vi "HFRR ADV v011 new software.vi"() -> ()   [LabVIEW 2025] (continued)
        n3525 = Unbundle By Name(w4415) -> ("Heave COM Status 2"=→"COM Status" →"Instrument Status":bool, "Error Heave"=→"Error":errorcluster)  [unwired: 1 out]
        n3526 = Bundle By Name(cluster=w4415, "LastCom"=w4413) -> (w4414:T18)
      }
      frame "MAIN" {
        n3527 = Unbundle By Name(w4438) -> ("Com Port 2"=w4450:refnum<visa-resource-name>)
        n3528 = local write "Com Port 4"(w4450) -> ()
        n3529 = local read "C3 :"() -> (w4436:refnum<visa-resource-name>)
        n3530 = Bundle By Name(cluster=w4438, "Heave and Surge COM Port:"=w4436) -> (w4437:T18)
        n3531 = Equal?(x=w4450, y=w4436) -> (x = y?=w4449:bool)
        n3532 = case shown="True" w4449 {
          tunnel: [w4454 w4471] -> w4448
          tunnel: w4439 -> [w4455 w4477]
          tunnel: w4437 -> [w4453 w4475]
          tunnel: [w4452 w4470] -> w4445
          frame False {
            n3533 = call <vilib>:"Clear Errors.vi"("error in (no error)"=w4455) -> ("error out"=w4451:errorcluster)  [unwired: 5 in, 1 out]
            n3534 = call "Instrument fgv.vi"("Enum"=T30."ERROR INIT", "error in (no error) 2"=w4451, "INPUT"=w4453) -> ("error"=w4457:errorcluster, "output"=w4452:T18)  [unwired: 6 in, 1 out]
            n3535 = call <vilib>:"Clear Errors.vi"("error in (no error)"=w4457) -> ("error out"=w4454:errorcluster)  [unwired: 5 in, 1 out]
          }
          frame True {
            n3536 = call "Instrument fgv.vi"("Enum"=T30."READ", "error in (no error) 2"=w4477, "INPUT"=w4475) -> ("error"=w4476:errorcluster, "output"=w4467:T18)  [unwired: 6 in, 1 out]
            n3537 = Bundle By Name(cluster=w4467, "String 36"="String 11") -> (w4466:T18)
            n3538 = case shown="True" "Write S" {
              selector: "Write S" -> [_ w4497]
              tunnel: w4476 -> [w4490 w4496]
              tunnel: [w4490 w4495] -> w4463
              tunnel: w4466 -> [w4489 w4492]
              tunnel: [w4489 w4491] -> w4462
              frame False {
              }
              frame True {
                n3539 = Not(x=w4497) -> (.not. x?=w4493:bool)
                n3540 = local write "Write S"(w4493) -> ()
                n3541 = call "Instrument fgv.vi"("Enum"=T30."MANUAL WRITE", "error in (no error) 2"=w4496, "INPUT"=w4492) -> ("error"=w4495:errorcluster, "output"=w4491:T18)  [unwired: 6 in, 1 out]
              }
            }
            n3542 = Array Size(array="WriteHumidity") -> (size(s)=w4460:i32)
            n3543 = Greater Than 0?(x=w4460) -> (x > 0?=w4458:bool)
            n3544 = call "Instrument fgv.vi"("Enum"=T30."WRITE", "error in (no error) 2"=w4463, "WriteCC1"="WriteHumidity", "INPUT"=w4462) -> ("error"=w4473:errorcluster, "WriteCC1 2"=w4461:string[], "output"=w4472:T18)  [unwired: 5 in]
            n3545 = case shown="True" w4458 {
              tunnel: w4461 -> [_ w4479]
              frame False {
              }
              frame True {
                n3546 = local write "WriteHumidity"(w4479) -> ()
              }
            }
            n3547 = case shown="Error" w4473 {
              selector: w4473 -> [w4480 w4483]
              tunnel: w4472 -> [w4481 w4488]
              tunnel: [w4481 w4487] -> w4470
              tunnel: [w4480 w4485] -> w4471
              frame No Error {
              }
              frame Error {
                n3548 = call <vilib>:"Clear Errors.vi"("error in (no error)"=w4483) -> ("error out"=w4482:errorcluster)  [unwired: 5 in, 1 out]
                n3549 = call "Instrument fgv.vi"("Enum"=T30."ERROR INIT", "error in (no error) 2"=w4482, "INPUT"=w4488) -> ("error"=w4486:errorcluster, "output"=w4487:T18)  [unwired: 6 in, 1 out]
                n3550 = call <vilib>:"Clear Errors.vi"("error in (no error)"=w4486) -> ("error out"=w4485:errorcluster)  [unwired: 5 in, 1 out]
              }
            }
            n3551 = Unbundle By Name(w4470) -> ("LastCom"=→"LastCom":string, "Read Heave and Surge"=→"Read Humidity":string)
          }
        }
        n3552 = Unbundle By Name(w4445) -> ("Heave COM Status 2"=w4447:bool, "Heave COM Status"=w4446:bool, "Error Heave"=w4443:errorcluster, "Bytes at Heave Port"=→"Bytes at Humidity Port":dbl)
        n3553 = Unbundle By Name(w4443) -> ("status"=→"Humidity Port":bool)
        n3554 = Not(x=w4446) -> (.not. x?=w4440:bool)
        n3555 = local write "Error"(w4443) -> ()
        n3556 = Not(x=w4447) -> (.not. x?=w4441:bool)
        n3557 = local write "Instrument Status"(w4440) -> ()
        n3558 = local write "COM Status"(w4441) -> ()
        n3559 = local read "Quit"() -> (w4433:bool)
        n3560 = Select(t=enum16{"init", "MAIN", "Panel Close"}."Panel Close", s=w4433, f=enum16{"init", "MAIN", "Panel Close"}."MAIN") -> (s? t:f=w4432:enum16{"init", "MAIN", "Panel Close"})
      }
      frame "Panel Close" {
      }
      frame Default {
      }
    }
  }
  n3561 = while {
    stop <- w4528 stop-if-true
    n3562 = local read "Read Humidity"() -> (w4509:string)
    n3563 = call <vilib>:"High Resolution Polling Wait.vi"("seconds to wait"=0.1) -> ()  [unwired: 10 in, 1 out]
    n3564 = Spreadsheet String To Array(delimiter (Tab)=",", format string="", spreadsheet string=w4509, array type (2D Dbl)=string[] []) -> (array=w4523:string[])
    n3565 = for {
      tunnel: w4523 -> [w4533] mode=indexing
      tunnel: string[] ["STATE;", "SET;", "RH;", "T;", "AMB_RH;", "AMB_T;", "PUMP;", "FAN_IN;", "FAN_OUT;", "DEHUM;", "CURRENT;", "STALL;"] -> [w4532] mode=indexing
      tunnel: [w4531] -> w4522 mode=indexing
      n3566 = Match Pattern(string=w4533, regular expression=w4532) -> (after substring=w4531:string)  [unwired: 1 in, 3 out]
    }
    n3567 = Index Array(array=w4522) -> (element #1=→"STATE :":string, element #2=→"SET :":string, element #3=w4511:string, element #4=→"T :":string, element #5=w4508:string, element #6=→"AMB_T :":string, element #7=→"PUMP :":string, element #8=→"FAN_IN :":string, element #9=→"FAN_OUT :":string, element #10=→"DEHUM :":string, element #11=→"CURRENT :":string, element #12=→"STALL :":string)  [unwired: 12 in]
    "RH :" <- w4511
    "AMB_RH :" <- w4508
    n3568 = Fract/Exp String To Number(string=w4511) -> (number=w4503:dbl)  [unwired: 3 in, 1 out]
    n3569 = Fract/Exp String To Number(string=w4508) -> (number=w4507:dbl)  [unwired: 3 in, 1 out]
    n3570 = local write "Ambient Humidity :"(w4507) -> ()
    n3571 = Equal?(x=w4503, y=0.0) -> (x = y?=w4505:bool)
    n3572 = case shown="True" w4505 {
      tunnel: [w4529 w4530] -> w4504
      tunnel: w4503 -> [w4529 _]
      frame False {
        (unwired) 0.0
        "Humidity temp" <- w4529
      }
      frame True {
        n3573 = local read "Humidity temp"() -> (w4530:dbl)
      }
    }
    "RH Numeric:" <- w4504
    n3574 = local read "Quit"() -> (w4528:bool)
  }
  n3575 = disable-structure shown="Disabled" {
    frame Disabled {
      n3576 = while {
        tunnel: [w4767] -> _
        i -> [w4767]
        stop <- w4764 stop-if-true
        n3577 = local read "powstat"() -> (w4765:bool)
        n3578 = case shown="True" w4765 {
          frame False {
          }
          frame True {
            n3579 = local read "RUN"() -> (w4768:bool)
            n3580 = case shown="True" w4768 {
              frame False {
                w4798 = 65.0 ("y")
                n3581 = local read "Set Hz"() -> (w4826:dbl)
                n3582 = local read "NORMAL LOAD"() -> (w4827:dbl)
                n3583 = Multiply(x=w4826, y=60.0) -> (x*y=w4833:dbl)
                n3584 = Multiply(x=1.2 ("y"), y=0.949) -> (x*y=w4802:dbl)
                n3585 = Multiply(x=1.2 ("y"), y=0.8166) -> (x*y=w4806:dbl)
                n3586 = Multiply(x=1.2 ("y"), y=0.851) -> (x*y=w4801:dbl)
                n3587 = local read "FF 2"() -> (w4825:dbl)
                n3588 = Absolute Value(x=w4833) -> (abs(x)=w4831:dbl)
                n3589 = case shown="13.." w4825 {
                  tunnel: [1 2 3] -> w4823
                  frame 0..10, Default {
                    # "Normal"
                  }
                  frame 11, 12 {
                  }
                  frame 13.. {
                  }
                }
                "FF STATE" <- w4823
                n3590 = local read "TEMP"() -> (w4786:dbl)
                n3591 = local read item#-1() -> (w4800)
                n3592 = Less?(x=w4800, y=w4806) -> (x < y?=w4803:bool)
                n3593 = In Range and Coerce(upper limit=w4802, x=w4800, lower limit=w4801) -> (In Range?=w4804:bool)  [unwired: 1 out]
                n3594 = case shown="3601.." w4831 {
                  tunnel: [1 2 3] -> w4829
                  frame 0..3000, Default {
                    # "Normal"
                  }
                  frame 3001..3600 {
                  }
                  frame 3601.. {
                  }
                }
                n3595 = case shown="11.." w4827 {
                  tunnel: [1 3] -> w4828
                  frame 1..10, Default {
                  }
                  frame 11.. {
                  }
                }
                "NL STATE" <- w4828
                n3596 = Multiply(x=1.2 ("y"), y=0.95) -> (x*y=w4816:dbl)
                n3597 = Multiply(x=w4798, y=0.954) -> (x*y=w4790:dbl)
                n3598 = Or(x=w4803, y=w4804) -> (x .or. y?=w4805:bool)
                n3599 = Greater Or Equal?(x=w4800, y=w4816) -> (x >= y?=w4813:bool)
                n3600 = Multiply(x=w4798, y=0.99) -> (x*y=w4787:dbl)
                n3601 = Greater Or Equal?(x=w4786, y=w4787) -> (x >= y?=w4792:bool)
                n3602 = Greater Or Equal?(x=w4786, y=w4790) -> (x >= y?=w4789:bool)
                n3603 = case shown="0, 1, Default" w4800 {
                  tunnel: [1 3] -> w4817
                  frame 0, 1, Default {
                  }
                  frame 2.. {
                  }
                }
                n3604 = case shown="True" w4813 {
                  tunnel: [1 3] -> w4818
                  frame False {
                  }
                  frame True {
                  }
                }
                n3605 = case shown="True" w4805 {
                  tunnel: [1 2] -> w4819
                  frame False {
                  }
                  frame True {
                  }
                }
                n3606 = case shown="..0" w4786 {
                  tunnel: [2 3 3 1] -> w4793
                  frame 61, 62 {
                  }
                  frame 63.. {
                  }
                  frame ..0 {
                  }
                  frame 10..60, Default {
                  }
                }
                n3607 = case shown="True" w4792 {
                  tunnel: [1 3] -> w4794
                  frame False {
                  }
                  frame True {
                  }
                }
                n3608 = Number To Decimal String(number=w4829) -> (decimal integer string=w4830:string)  [unwired: 1 in]
                n3609 = case shown="True" w4789 {
                  tunnel: [1 2] -> w4795
                  frame False {
                  }
                  frame True {
                  }
                }
                n3610 = Number To Decimal String(number=1) -> (decimal integer string=→"Air temp":string)  [unwired: 1 in]
                n3611 = Number To Decimal String(number=w4823) -> (decimal integer string=→"ff_st":string)  [unwired: 1 in]
                n3612 = local write "sp_st"(w4830) -> ()
                n3613 = Number To Decimal String(number=w4828) -> (decimal integer string=→"nl_st":string)  [unwired: 1 in]
                n3614 = Build Array(w4793, w4794, w4795) -> (w4796:i32[])
                n3615 = Build Array(w4817, w4818, w4819) -> (w4820:i32[])
                n3616 = Array Max & Min(array=w4796) -> (max value=w4797:i32)  [unwired: 3 out]
                n3617 = Array Max & Min(array=w4820) -> (max value=w4821:i32)  [unwired: 3 out]
                n3618 = Number To Decimal String(number=w4797) -> (decimal integer string=w4785:string)  [unwired: 1 in]
                n3619 = Number To Decimal String(number=w4821) -> (decimal integer string=→"Stroke Ln 2":string)  [unwired: 1 in]
                n3620 = local write "temp_st"(w4785) -> ()
              }
              frame True {
                w4883 = 65.0 ("y")
                # "Healthy -1\nWarning -2\nError -3"
                n3621 = local read "TEMP"() -> (w4894:dbl)
                n3622 = local read "NORMAL LOAD"() -> (w4898:dbl)
                n3623 = local read "Set Hz"() -> (w4896:dbl)
                n3624 = Multiply(x=1.2 ("y"), y=0.949) -> (x*y=w4878:dbl)
                n3625 = Multiply(x=1.2 ("y"), y=0.8166) -> (x*y=w4874:dbl)
                n3626 = Multiply(x=1.2 ("y"), y=0.851) -> (x*y=w4879:dbl)
                n3627 = Multiply(x=w4883, y=0.954) -> (x*y=w4890:dbl)
                n3628 = Multiply(x=w4883, y=0.99) -> (x*y=w4893:dbl)
                n3629 = Greater Or Equal?(x=w4894, y=w4893) -> (x >= y?=w4888:bool)
                n3630 = Multiply(x=w4896, y=60.0) -> (x*y=w4902:dbl)
                n3631 = Greater Or Equal?(x=w4894, y=w4890) -> (x >= y?=w4891:bool)
                n3632 = local read "FF 2"() -> (w4897:dbl)
                n3633 = local read item#-1() -> (w4880)
                n3634 = Less?(x=w4880, y=w4874) -> (x < y?=w4877:bool)
                n3635 = In Range and Coerce(upper limit=w4878, x=w4880, lower limit=w4879) -> (In Range?=w4876:bool)  [unwired: 1 out]
                n3636 = Absolute Value(x=w4902) -> (abs(x)=w4900:dbl)
                n3637 = case shown="63.." w4894 {
                  tunnel: [2 3 3 1] -> w4887
                  frame 61, 62 {
                  }
                  frame 63.. {
                  }
                  frame ..0 {
                  }
                  frame 10..60, Default {
                  }
                }
                n3638 = case shown="True" w4888 {
                  tunnel: [1 3] -> w4886
                  frame False {
                  }
                  frame True {
                  }
                }
                n3639 = case shown="True" w4891 {
                  tunnel: [1 2] -> w4885
                  frame False {
                  }
                  frame True {
                  }
                }
                n3640 = Multiply(x=1.2 ("y"), y=0.95) -> (x*y=w4864:dbl)
                n3641 = case shown="1..10, Default" w4898 {
                  tunnel: [1 3] -> w4905
                  frame 1..10, Default {
                  }
                  frame 11.. {
                  }
                }
                n3642 = case shown="0..10, Default" w4897 {
                  tunnel: [1 2 3] -> w4904
                  frame 0..10, Default {
                  }
                  frame 11, 12 {
                  }
                  frame 13.. {
                  }
                }
                n3643 = case shown="3601.." w4900 {
                  tunnel: [1 2 3] -> w4899
                  frame 0..3000, Default {
                    # "Normal"
                  }
                  frame 3001..3600 {
                  }
                  frame 3601.. {
                  }
                }
                n3644 = Or(x=w4877, y=w4876) -> (x .or. y?=w4875:bool)
                n3645 = Greater Or Equal?(x=w4880, y=w4864) -> (x >= y?=w4867:bool)
                n3646 = case shown="0, 1, Default" w4880 {
                  tunnel: [1 3] -> w4863
                  frame 0, 1, Default {
                  }
                  frame 2.. {
                  }
                }
                n3647 = case shown="True" w4867 {
                  tunnel: [1 3] -> w4862
                  frame False {
                  }
                  frame True {
                  }
                }
                n3648 = case shown="True" w4875 {
                  tunnel: [1 2] -> w4861
                  frame False {
                  }
                  frame True {
                  }
                }
                n3649 = Build Array(w4887, w4886, w4885) -> (w4884:i32[])
                n3650 = Number To Decimal String(number=w4899) -> (decimal integer string=→"sp_st":string)  [unwired: 1 in]
                n3651 = Array Max & Min(array=w4884) -> (max value=w4881:i32)  [unwired: 3 out]
                "TEMP STATE" <- w4881
                n3652 = Number To Decimal String(number=w4905) -> (decimal integer string=w4908:string)  [unwired: 1 in]
                n3653 = Number To Decimal String(number=w4904) -> (decimal integer string=w4906:string)  [unwired: 1 in]
                n3654 = Number To Decimal String(number=w4881) -> (decimal integer string=→"temp_st":string)  [unwired: 1 in]
                n3655 = Build Array(w4863, w4862, w4861) -> (w4860:i32[])
                n3656 = local write "nl_st"(w4908) -> ()
                n3657 = local write "ff_st"(w4906) -> ()
                n3658 = Number To Decimal String(number=1) -> (decimal integer string=w4903:string)  [unwired: 1 in]
                n3659 = Array Max & Min(array=w4860) -> (max value=w4859:i32)  [unwired: 3 out]
                n3660 = local write "Air temp"(w4903) -> ()
                n3661 = Number To Decimal String(number=w4859) -> (decimal integer string=w4858:string)  [unwired: 1 in]
                n3662 = local write "Stroke Ln 2"(w4858) -> ()
              }
            }
            n3663 = local read "Stroke Ln 2"() -> (w4770:string)
            n3664 = local read "nl_st"() -> (w4776:string)
            n3665 = local read "ff_st"() -> (w4773:string)
            n3666 = local read "sp_st"() -> (w4774:string)
            n3667 = local read "temp_st"() -> (w4775:string)
            n3668 = local read "Air temp"() -> (w4769:string)
            n3669 = Replace Array Subset(array="in", new element #1=w4776, index #1=1 ("index"), new element #2=w4773, index #2=2 ("index"), new element #3=w4775, index #3=3 ("index"), new element #4=w4774, index #4=4 ("index"), new element #5=w4770, index #5=5 ("index"), new element #6=w4769, index #6=6 ("index"), new element #7="Sensor State" ("new element/subarray"), index #7=0 ("index")) -> (→"out":string[])
          }
        }
        n3670 = Wait (ms)(milliseconds to wait=u32 10) -> ()  [unwired: 1 out]
        n3671 = local read "Quit"() -> (w4764:bool)
      }
      n3672 = while {
        stop <- w4739 stop-if-true
        n3673 = local read "run replace"() -> (w4741:bool)
        n3674 = Wait (ms)(milliseconds to wait=u32 100) -> ()  [unwired: 1 out]
        n3675 = Equal?(x="FLAG 2", y=0.0) -> (x = y?=w4742:bool)
        n3676 = case shown="True" w4742 {
          frame False {
          }
          frame True {
            n3677 = local write "FLAG 2"(100.0 ("FLAG 2")) -> ()
            n3678 = call <vilib>:"Read Characters From File.vi"("file path (dialog if empty)"=path "C:/LAB-IQ-NXT/WO 2449 TT.sig", "convert eol? (no:F)"=FALSE ("append to file? (new file:F)")) -> ("character string"=w4745:string)  [unwired: 4 in, 3 out]
            n3679 = call <vilib>:"Read Characters From File.vi"("file path (dialog if empty)"=path "C:/LAB-IQ-NXT/WO 2449 TRH.sig", "convert eol? (no:F)"=FALSE ("append to file? (new file:F)")) -> ("character string"=w4746:string)  [unwired: 4 in, 3 out]
            n3680 = Decimal String To Number(string=w4745) -> (number=w4747:i32)  [unwired: 2 in, 1 out]
            n3681 = local write "Total No. of Tests"(w4747) -> ()
            n3682 = Decimal String To Number(string=w4746) -> (number=w4750:i32)  [unwired: 2 in, 1 out]
            n3683 = local write "SEN.RUN HRS"(w4750) -> ()
          }
        }
        n3684 = case shown="True" w4741 {
          frame False {
          }
          frame True {
            n3685 = Equal?(x="FLAG 4", y=0.0) -> (x = y?=w4754:bool)
            n3686 = case shown="False" w4754 {
              frame False {
                n3687 = Get Date/Time In Seconds() -> (seconds since 1Jan1904=w4760:timestamp)
                n3688 = local read "START 3"() -> (w4758:dbl)
                n3689 = To Double Precision Float(number=w4760) -> (double precision float=w4759:dbl)
                n3690 = Subtract(x=w4759, y=w4758) -> (x-y=→"SENSOR TIME":dbl)
              }
              frame True {
                n3691 = Get Date/Time In Seconds() -> (seconds since 1Jan1904=w4762:timestamp)
                n3692 = local write "FLAG 4"(100.0 ("FLAG")) -> ()
                n3693 = To Double Precision Float(number=w4762) -> (double precision float=→"START 3":dbl)
              }
            }
          }
        }
        n3694 = local read "Quit"() -> (w4739:bool)
      }
      n3695 = while {
        shift-right: [w4539] -> _
        shift-left: _ -> [w4540]
        tunnel: [w4535] -> _
        i -> [w4535]
        stop <- w4534 stop-if-true
        n3696 = Wait (ms)(milliseconds to wait=u32 50 ("Refresh Rate (ms)")) -> ()  [unwired: 1 out]
        n3697 = local read "Json End Flg"() -> (w4536:bool)
        n3698 = Not(x="Upld AR 2") -> ()  [unwired: 1 out]
        n3699 = local read "Upld AR 2"() -> (w4537:bool)
        n3700 = call "Elapsed Time9"("Time Target (s)"="Sen.Upload Rate (s)", "Reset"=FALSE, "Auto Reset"=TRUE) -> ("Time has Elapsed"=w4546:bool)  [unwired: 9 in, 7 out]
        n3701 = Or(x=w4546, y=w4536) -> (x .or. y?=w4542:bool)
        n3702 = case shown="True" w4542 {
          frame False {
          }
          frame True {
            w4638 = "\"SensorName\":\"" ("string")
            w4608 = " \"},{"
            w4633 = "\",\"SensorState\":\""
            w4635 = "\",\"SensorModelNumber\":\"" ("string")
            w4634 = "\",\"SensorRuntimeHours\":\"" ("string")
            n3703 = local read "model num"() -> (w4632:string[])
            n3704 = local read "Sensor name"() -> (w4651:string[])
            n3705 = local read "run"() -> (w4622:string[])
            n3706 = local read "SENSOR TIME"() -> (w4578:dbl)
            n3707 = local read "out"() -> (w4571:string[])
            n3708 = local read "Total No. of Tests"() -> (w4576:dbl)
            n3709 = Select(t=60.0, s="Run test 3", f=3600.0) -> (s? t:f=w4586:dbl)
            n3710 = Index Array(array=w4632, index #1=1 ("index")) -> (element #1=w4631:string, element #2=w4630:string, element #3=w4629:string, element #4=w4628:string, element #5=w4627:string, element #6=w4626:string)  [unwired: 5 in]
            n3711 = Index Array(array=w4622, index #1=1 ("index")) -> (element #1=w4621:string, element #2=w4620:string, element #3=w4619:string, element #4=w4618:string, element #5=w4617:string, element #6=w4616:string)  [unwired: 5 in]
            n3712 = Index Array(array=w4651, index #1=1 ("index")) -> (element #1=w4650:string, element #2=w4649:string, element #3=w4648:string, element #4=w4647:string, element #5=w4637:string, element #6=w4636:string)  [unwired: 5 in]
            n3713 = Index Array(array=w4571, index #1=1 ("index")) -> (element #1=w4603:string, element #2=w4602:string, element #3=w4601:string, element #4=w4600:string, element #5=w4599:string, element #6=w4598:string)  [unwired: 5 in]
            n3714 = local read "SEN.RUN HRS"() -> (w4574:dbl)
            n3715 = Divide(x=w4578, y=w4586) -> (x/y=w4585:dbl)
            n3716 = Increment(x=w4585) -> (x+1=w4581:dbl)
            n3717 = Number To Decimal String(number=w4581) -> (decimal integer string=→"run hrs":string)  [unwired: 1 in]
            n3718 = Divide(x=w4574, y=3600.0 ("f")) -> (x/y=w4569:dbl)
            n3719 = Round To Nearest(number=w4569) -> (nearest integer value=w4567:dbl)
            n3720 = Number To Decimal String(number=w4567) -> (decimal integer string=w4568:string)  [unwired: 1 in]
            n3721 = Number To Decimal String(number=w4576) -> (decimal integer string=w4577:string)  [unwired: 1 in]
            n3722 = local read "Model No"() -> (w4582:string)
            n3723 = local read "UUID"() -> (w4677:string)
            n3724 = local read "Serial No"() -> (w4681:string)
            n3725 = local read "Secret Key"() -> (w4682:string)
            n3726 = Concatenate Strings("\",\"MachineSerialNumber\":\"" ("string"), w4681) -> (w4685:string)
            n3727 = Concatenate Strings("\",\"ModelNumber\":\"" ("string"), w4582) -> (w4583:string)
            n3728 = Concatenate Strings("\",\"MachineRuntimeHours\":\"" ("string"), w4568) -> (w4686:string)
            n3729 = Concatenate Strings("\",\"MachineRuntimeCycles\":\"", w4577) -> (w4679:string)
            n3730 = Concatenate Strings(w4635, w4631) -> (w4665:string)
            n3731 = Concatenate Strings(w4634, w4621) -> (w4666:string)
            n3732 = Concatenate Strings(w4633, w4603) -> (w4664:string)
            n3733 = Concatenate Strings(w4685, w4583, w4686, w4679) -> (w4688:string)
            n3734 = Concatenate Strings(w4635, w4630) -> (w4662:string)
            n3735 = Concatenate Strings(w4634, w4620) -> (w4661:string)
            n3736 = Concatenate Strings(w4633, w4602) -> (w4663:string)
            n3737 = Concatenate Strings(w4635, w4629) -> (w4657:string)
            n3738 = Concatenate Strings(w4634, w4619) -> (w4658:string)
            n3739 = Concatenate Strings(w4633, w4601) -> (w4656:string)
            n3740 = Concatenate Strings(w4635, w4628) -> (w4654:string)
            n3741 = Concatenate Strings(w4634, w4618) -> (w4653:string)
            n3742 = Concatenate Strings(w4633, w4600) -> (w4655:string)
            n3743 = Concatenate Strings(w4665, w4666, w4664) -> (w4667:string)
            n3744 = Concatenate Strings(w4635, w4627) -> (w4644:string)
            n3745 = Concatenate Strings(w4634, w4617) -> (w4645:string)
            n3746 = Concatenate Strings(w4635, w4626) -> (w4641:string)
            n3747 = Concatenate Strings(w4634, w4616) -> (w4640:string)
            n3748 = Concatenate Strings(w4633, w4599) -> (w4643:string)
            n3749 = Concatenate Strings(w4633, w4598) -> (w4642:string)
            n3750 = Concatenate Strings("{\"SecretKey\":\"", w4682, w4688, "\",\"UUID\" : \"", w4677, "\",\"SensorInformation\":", "[{" ("string")) -> (w4615:string)
            n3751 = Concatenate Strings(w4662, w4661, w4663) -> (w4660:string)
            n3752 = Concatenate Strings(w4657, w4658, w4656) -> (w4659:string)
            n3753 = Concatenate Strings(w4654, w4653, w4655) -> (w4652:string)
            n3754 = Concatenate Strings(w4644, w4645, w4643) -> (w4646:string)
            n3755 = Concatenate Strings(w4641, w4640, w4642) -> (w4639:string)
            n3756 = Concatenate Strings(w4638, w4650, w4667, w4608) -> (w4614:string)
            n3757 = Concatenate Strings(w4638, w4649, w4660, w4608) -> (w4613:string)
            n3758 = Concatenate Strings(w4638, w4648, w4659, w4608) -> (w4612:string)
            n3759 = Concatenate Strings(w4638, w4647, w4652, w4608) -> (w4611:string)
            n3760 = Concatenate Strings(w4638, w4637, w4646, w4608) -> (w4610:string)
            n3761 = Concatenate Strings(w4638, w4636, w4639, "\"}" ("string")) -> (w4609:string)
            n3762 = Concatenate Strings(w4615, w4614, w4613, w4612, w4611, w4610, w4609, "]}" ("string")) -> (w4606:string)
            n3763 = local read "SEN.RUN HRS"() -> (w4573:dbl)
            n3764 = disable-structure shown="Disabled" {
              frame Disabled {
                n3765 = local read "state"() -> (w4692:string[])
                n3766 = Delete From Array(array=w4692, index=0) -> (array with subset deleted=w4690:string[])  [unwired: 1 in, 1 out]
                n3767 = for {
                  N: 6 -> [_]
                  tunnel: w4690 -> [w4703] mode=indexing
                  tunnel: [w4702] -> w4689 mode=indexing
                  n3768 = Equal?(x=w4703, y="Warning") -> (x = y?=w4699:bool)
                  n3769 = Equal?(x=w4703, y="Healthy") -> (x = y?=w4696:bool)
                  n3770 = Select(t="2" ("y"), s=w4699, f="3" ("y")) -> (s? t:f=w4694:string)
                  n3771 = Select(t="1" ("y"), s=w4696, f=w4694) -> (s? t:f=w4702:string)
                }
                "state1" <- w4689
              }
              frame Enabled {
              }
            }
            n3772 = stacked-sequence {
              tunnel: w4606 -> [w4714 _ _]
              tunnel: [_ _ w4730] -> _
              frame #0 {
                (unwired) FALSE ("convert eol (F)")
                w4716 = enum16{"start", "end", "current"}."start" ("pos mode (0:2)")
                n3773 = local read "Path"() -> (w4710:path)
                n3774 = Path To String(path=w4710) -> (string=w4722:string)
                n3775 = Concatenate Strings(w4722, "\\", "Sensor File Name") -> (w4723:string)
                n3776 = local write "standard output 2"(" ") -> ()
                n3777 = String To Path(string=w4723) -> (path=w4713:path)
                n3778 = call <vilib>:"Open_Create_Replace File.vi"("advisory dialog? (display:T)"=FALSE, "function (open:0)"=T31."create or replace", "file path"=w4713) -> ("error out"=w4726:errorcluster, "refnum"=w4725:refnum<file>)  [unwired: 5 in, 2 out]
                n3779 = Set File Position(refnum=w4725, from (0:start)=w4716, error in=w4726) -> (refnum out=w4706:refnum<file>, error out=w4705:errorcluster)  [unwired: 1 in]
                n3780 = Write to Binary File(file (use dialog)=w4706, data=" ", error in=w4705, 5:FALSE ("prepend array or string size? (T)")) -> (refnum out=w4717:refnum<file>, error out=w4718:errorcluster)  [unwired: 2 in, 1 out]
                n3781 = Set File Position(offset (in bytes) (0)=w4716, refnum=w4717, error in=w4718) -> (refnum out=w4709:refnum<file>, error out=w4708:errorcluster)  [unwired: 1 in]
                n3782 = Write to Binary File(file (use dialog)=w4709, data=w4714, error in=w4708, 5:FALSE ("prepend array or string size? (T)")) -> (error out=w4712:errorcluster)  [unwired: 2 in, 2 out]
                n3783 = flat-sequence {
                  tunnel: w4713 -> [w4728]
                  tunnel: w4712 -> [_]
                  frame #0 {
                    n3784 = call <vilib>:"Read Characters From File.vi"("file path (dialog if empty)"=w4728) -> ("character string"=→"Sensor Health JSON string":string)  [unwired: 5 in, 3 out]
                  }
                }
                "SinglePoint  2" <- w4714
              }
              frame #1 {
              }
              frame #2 {
                (unwired) "\"Stored\": true" ("string")
                n3785 = call <vilib>:"System Exec.vi"("run minimized? (F)"=TRUE, "wait until completion? (T)"=TRUE, "working directory"=path "C:/LAB-IQ-NXT", "command line"="C:\\LAB-IQ-NXT\\JPostH.bat") -> ("standard error"=→"Respose From Server 2":string, "standard output"=w4733:string)  [unwired: 4 in, 2 out]
                "standard output 2" <- w4733
                n3786 = Match Pattern(string=w4733, regular expression="JSONH Check String") -> (match substring=w4731:string, offset past match=w4730:i32)  [unwired: 1 in, 2 out]
                n3787 = Equal?(x=w4731, y="JSONH Check String") -> (x = y?=→"Upload \nConfirmed 2":bool)
              }
            }
            n3788 = Divide(x=w4573, y=3600.0 ("f")) -> (x/y=w4566:dbl)
            n3789 = local read "run time"() -> (w4623:string[])
            n3790 = Round To Nearest(number=w4566) -> (nearest integer value=w4565:dbl)
            n3791 = Number To Decimal String(number=w4565) -> (decimal integer string=w4564:string)  [unwired: 1 in]
            n3792 = Index Array(array="Sensor Information", index (col) #1=0 ("disabled index (col)"), index (col) #2=1 ("index (col)"), index (col) #3=2 ("index (col)"), index (col) #4=3 ("index (col)")) -> (element #1=→"Sensor name":string[], element #2=→"model num":string[], element #3=→"run time":string[], element #4=→"state":string[])  [unwired: 4 in]
            n3793 = Insert Into Array(array=w4623, index=1, new element #1=w4564, new element #2=w4564, new element #3=w4564, new element #4=w4564, new element #5=w4564, new element #6=w4564) -> (w4588:string[])
            "run" <- w4588
            n3794 = local read "out"() -> (w4570:string[])
            n3795 = local read "Sensor Information"() -> (w4590:string[][])
            n3796 = Replace Array Subset(array=w4590, new element #1=w4588, index (col) #1=2 ("disabled index (col)"), new element #2=w4570, index (col) #2=3 ("index (col)")) -> (w4589:string[][])  [unwired: 2 in]
            n3797 = local write "Sensor Information"(w4589) -> ()
          }
        }
        n3798 = case shown="True" w4537 {
          frame False {
          }
          frame True {
            n3799 = Equal?(x="FLAG", y=0.0) -> (x = y?=w4554:bool)
            n3800 = case shown="False" w4554 {
              frame False {
                n3801 = Get Date/Time In Seconds() -> (seconds since 1Jan1904=w4560:timestamp)
                n3802 = local read "START 2"() -> (w4558:dbl)
                n3803 = To Double Precision Float(number=w4560) -> (double precision float=w4559:dbl)
                n3804 = Subtract(x=w4559, y=w4558) -> (x-y=→"SENSOR TIME  2":dbl)
              }
              frame True {
                n3805 = Get Date/Time In Seconds() -> (seconds since 1Jan1904=w4562:timestamp)
                n3806 = To Double Precision Float(number=w4562) -> (double precision float=→"START 2":dbl)
                n3807 = local write "FLAG"(100.0 ("FLAG")) -> ()
              }
            }
          }
        }
        n3808 = disable-structure shown="Disabled" {
          disable-tunnel: w4540 -> [w4549 _]
          disable-tunnel: [w4548 _] -> w4539
          frame Disabled {
            n3809 = local read "Json St Flg"() -> (w4547:bool)
            n3810 = case shown="True" w4547 {
              tunnel: w4549 -> [w4550 w4552]
              tunnel: [w4550 w4551] -> w4548
              frame False {
              }
              frame True {
                n3811 = Increment(x=w4552) -> (x+1=w4551:dbl)
                "T cycle" <- w4551
                n3812 = local write "Json St Flg"(FALSE ("Json St Flg")) -> ()
              }
            }
          }
          frame Enabled {
          }
        }
        n3813 = local read "Quit"() -> (w4534:bool)
      }
    }
    frame Enabled {
    }
  }
  n3814 = stacked-sequence {
    tunnel: [w4932] -> w38
    frame #0 {
      w4932 = FALSE ("Upload \nConfirmed")
      n3815 = local write "Upload \nConfirmed"(w4932) -> ()
      n3816 = local write "St Str"("") -> ()
    }
  }
  n3817 = disable-structure shown="Disabled" {
    disable-tunnel: w38 -> [w4933 _]
    frame Disabled {
      n3818 = case shown="True" {
        selector: _ -> [_ _]
        tunnel: w4933 -> [_ w4934]
        frame False {
        }
        frame True {
          n3819 = while {
            tunnel: [w4940] -> _
            tunnel: w4934 -> [_]
            i -> [w4940]
            stop <- w4935 stop-if-true
            n3820 = local read "Json End Flg"() -> (w4939:bool)
            n3821 = Wait (ms)(milliseconds to wait=u32 20 ("Refresh Rate (ms)")) -> ()  [unwired: 1 out]
            n3822 = local read "refresh flag"() -> (w4936:bool)
            n3823 = local read "RUN"() -> (w4937:bool)
            n3824 = And(x=w4937, y=w4936) -> (x .and. y?=w4938:bool)
            n3825 = Or(x=w4938, y=w4939) -> (x .or. y?=w4941:bool)
            "AR Led" <- w4941
            n3826 = case shown="True" w4941 {
              frame False {
              }
              frame True {
                w4958 = "\",\""
                n3827 = local read "UUID"() -> (w4956:string)
                n3828 = local write "refresh flag"(FALSE ("refresh flag")) -> ()
                n3829 = local read "time"() -> (w4945:dbl)
                n3830 = Multiply(x=w4945, y=60.0) -> (x*y=w4944:dbl)
                n3831 = Concatenate Strings("UUID\" : \"", w4956, "\"}") -> (w4959:string)
                n3832 = Number To Fractional String(number=w4944, width (-)=i16 10, precision (6)=i16 4) -> (F-format string=w4973:string)  [unwired: 1 in]
                n3833 = Concatenate Strings("{", "\"Time\":\"", w4973, w4958) -> (w4968:string)
                n3834 = stacked-sequence {
                  tunnel: w4958 -> [w5021 w5029 w5036 w5044 w5052 w5061 w5068]
                  tunnel: [w5022 _ _ _ _ _ _] -> w4972
                  tunnel: [_ w5030 _ _ _ _ _] -> w4971
                  tunnel: [_ _ w5037 _ _ _ _] -> w4970
                  tunnel: [_ _ _ w5046 _ _ _] -> w4969
                  tunnel: w4959 -> [_ _ _ _ _ _ w5079]
                  tunnel: [_ _ _ _ _ _ w5078] -> w4955
                  tunnel: [_ _ _ _ _ w5058 _] -> w4954
                  tunnel: [_ _ _ _ w5051 _ _] -> w4953
                  frame #0 {
                    n3835 = local read "NORMAL LOAD"() -> (w5020:dbl)
                    n3836 = Number To Fractional String(number=w5020, width (-)=i16 10, precision (6)=i16 4) -> (F-format string=w5023:string)  [unwired: 1 in]
                    n3837 = Concatenate Strings("NormalLoad\":\"", w5023, w5021) -> (w5022:string)
                  }
                  frame #1 {
                    n3838 = local read "Temp"() -> (w5028:dbl)
                    n3839 = Number To Fractional String(number=w5028, width (-)=i16 10, precision (6)=i16 4) -> (F-format string=w5031:string)  [unwired: 1 in]
                    n3840 = Concatenate Strings("Temperature\":\"", w5031, w5029) -> (w5030:string)
                  }
                  frame #2 {
                    n3841 = local read "cof"() -> (w5034:dbl)
                    n3842 = Number To Fractional String(number=w5034, width (-)=i16 10, precision (6)=i16 4) -> (F-format string=w5038:string)  [unwired: 1 in]
                    n3843 = Concatenate Strings("FrictionalForce\":\"", w5038, w5036) -> (w5037:string)
                  }
                  frame #3 {
                    n3844 = local read "Set Hz"() -> (w5042:dbl)
                    n3845 = Multiply(x=w5042, y=60.0) -> (x*y=w5041:dbl)
                    n3846 = Number To Fractional String(number=w5041, width (-)=i16 10, precision (6)=i16 4) -> (F-format string=w5047:string)  [unwired: 1 in]
                    n3847 = Concatenate Strings("Speed\":\"", w5047, w5044) -> (w5046:string)
                  }
                  frame #4 {
                    n3848 = local read item#-1() -> (w5050)
                    n3849 = Number To Fractional String(number=w5050, width (-)=i16 10, precision (6)=i16 4) -> (F-format string=w5054:string)  [unwired: 1 in]
                    n3850 = Concatenate Strings("LinearDeformation\":\"", w5054, w5052) -> (w5051:string)
                  }
                  frame #5 {
                    n3851 = local read "AIR TEMP"() -> (w5057:dbl)
                    n3852 = local read "Json St Flg"() -> (w5059:bool)
                    n3853 = local read "Json End Flg"() -> (w5060:bool)
                    n3854 = Number To Fractional String(number=w5057, width (-)=i16 10, precision (6)=i16 4) -> (F-format string=w5063:string)  [unwired: 1 in]
                    n3855 = Concatenate Strings("Vibration\":\"", w5063, w5061) -> (w5058:string)
                    n3856 = And(x=w5059, y=w5060) -> ()  [unwired: 1 out]
                  }
                  frame #6 {
                    n3857 = local read "Json End Flg"() -> (w5067:bool)
                    n3858 = Get Date/Time In Seconds() -> (seconds since 1Jan1904=w5075:timestamp)
                    n3859 = local read "Json St Flg"() -> (w5066:bool)
                    n3860 = To Double Precision Float(number=w5075) -> (double precision float=w5074:dbl)
                    n3861 = Subtract(x=w5074, y=2082844800.0) -> (x-y=w5072:dbl)
                    n3862 = Number To Fractional String(number=w5072, width (-)=i16 12, precision (6)=i16 0) -> (F-format string=w5069:string)  [unwired: 1 in]
                    n3863 = case shown="True" w5067 {
                      tunnel: ["" w5082] -> w5076
                      tunnel: w5069 -> [_ w5083]
                      tunnel: w5068 -> [_ w5081]
                      frame False {
                      }
                      frame True {
                        n3864 = local write "Json End Flg"(FALSE ("Json St Flg")) -> ()
                        n3865 = Concatenate Strings("End\": \"", w5083, w5081) -> (w5082:string)
                      }
                    }
                    n3866 = case shown="True" w5066 {
                      tunnel: [w5086 w5089] -> w5077
                      tunnel: w5069 -> [_ w5090]
                      tunnel: w5068 -> [_ w5087]
                      frame False {
                        n3867 = local read "St Str"() -> (w5086:string)
                      }
                      frame True {
                        n3868 = Concatenate Strings("Start\":\"", w5090, w5087) -> (w5089:string)
                        "St Str" <- w5089
                        n3869 = local write "Json St Flg"(FALSE ("Json St Flg")) -> ()
                      }
                    }
                    n3870 = Concatenate Strings(w5077, w5076, w5079) -> (w5078:string)
                  }
                }
                n3871 = local read "FILE"() -> (w4947:string)
                n3872 = Concatenate Strings("\",\"OperatorID\":\"" ("string"), "Operator ID") -> (w4950:string)
                n3873 = Concatenate Strings("\",\"DatasetTitle\":\"" ("string"), w4947) -> (w4949:string)
                n3874 = Concatenate Strings("\",\"SerialNumber\":\"" ("string"), "Serial No") -> (w4979:string)
                n3875 = Concatenate Strings("\",\"ModelNumber\":\"" ("string"), "Model No") -> (w4978:string)
                n3876 = Concatenate Strings(w4979, w4978) -> (w4961:string)
                n3877 = Concatenate Strings("{\"SecretKey\":\"", "Secret Key", w4961, w4950, w4949, "\",\"Samples\":[") -> (w4966:string)
                n3878 = Concatenate Strings(w4968, w4972, w4971, w4970, w4969, w4953, w4954, w4955) -> (w4967:string)
                n3879 = Concatenate Strings(w4966, w4967, "]}") -> (w4965:string)
                n3880 = stacked-sequence {
                  tunnel: w4965 -> [w4994 _ _]
                  tunnel: [_ _ w5011] -> _
                  frame #0 {
                    (unwired) FALSE ("convert eol (F)")
                    w4996 = enum16{"start", "end", "current"}."start" ("pos mode (0:2)")
                    n3881 = Path To String(path="Path") -> (string=w5002:string)
                    n3882 = Concatenate Strings(w5002, "\\", "Data File Name") -> (w5004:string)
                    n3883 = local write "standard output"(" ") -> ()
                    n3884 = String To Path(string=w5004) -> (path=w4993:path)
                    n3885 = call <vilib>:"Open_Create_Replace File.vi"("advisory dialog? (display:T)"=FALSE, "function (open:0)"=T31."create or replace", "file path"=w4993) -> ("error out"=w5007:errorcluster, "refnum"=w5006:refnum<file>)  [unwired: 5 in, 2 out]
                    n3886 = Set File Position(refnum=w5006, from (0:start)=w4996, error in=w5007) -> (refnum out=w4987:refnum<file>, error out=w4986:errorcluster)  [unwired: 1 in]
                    n3887 = Write to Binary File(file (use dialog)=w4987, data=" ", error in=w4986, 5:FALSE ("prepend array or string size? (T)")) -> (refnum out=w4997:refnum<file>, error out=w4998:errorcluster)  [unwired: 2 in, 1 out]
                    n3888 = Set File Position(offset (in bytes) (0)=w4996, refnum=w4997, error in=w4998) -> (refnum out=w4990:refnum<file>, error out=w4989:errorcluster)  [unwired: 1 in]
                    n3889 = Write to Binary File(file (use dialog)=w4990, data=w4994, error in=w4989, 5:FALSE ("prepend array or string size? (T)")) -> (error out=w4992:errorcluster)  [unwired: 2 in, 2 out]
                    n3890 = flat-sequence {
                      tunnel: w4993 -> [w5009]
                      tunnel: w4992 -> [_]
                      frame #0 {
                        n3891 = call <vilib>:"Read Characters From File.vi"("file path (dialog if empty)"=w5009) -> ("character string"=→"JSON string":string)  [unwired: 5 in, 3 out]
                      }
                    }
                    "SinglePoint" <- w4994
                  }
                  frame #1 {
                  }
                  frame #2 {
                    (unwired) "\"Stored\": true" ("string")
                    n3892 = call <vilib>:"System Exec.vi"("run minimized? (F)"=TRUE, "wait until completion? (T)"=TRUE, "working directory"=path "C:/LAB-IQ-NXT", "command line"="C:\\LAB-IQ-NXT\\JPost.bat") -> ("standard error"=→"Respose From Server":string, "standard output"=w5014:string)  [unwired: 4 in, 2 out]
                    "standard output" <- w5014
                    n3893 = Match Pattern(string=w5014, regular expression="JSON Check String") -> (match substring=w5012:string, offset past match=w5011:i32)  [unwired: 1 in, 2 out]
                    n3894 = Equal?(x=w5012, y="JSON Check String") -> (x = y?=→"Upload \nConfirmed":bool)
                  }
                }
              }
            }
            n3895 = local read "Quit"() -> (w4935:bool)
          }
        }
      }
    }
    frame Enabled {
    }
  }
  n3896 = disable-structure shown="Disabled" {
    disable-tunnel: _ -> [w5097 _]
    frame Disabled {
      n3897 = while {
        shift-right: [w5105] -> w5093
        shift-left: _ -> [w5106]
        shift-right: [w5103] -> w5094
        shift-left: errorcluster {"status"=TRUE, "code"=0, "source"="Init"} ("error out") -> [w5104]
        shift-right: [w5101] -> _
        shift-left: "" -> [w5102]
        tunnel: [w5099] -> _
        tunnel: w5097 -> [_]
        i -> [w5099]
        stop <- w5098 stop-if-true
        n3898 = flat-sequence {
          tunnel: [w5107] -> w5100
          frame #0 {
            n3899 = Wait (ms)(milliseconds to wait=10.0 ("Delay")) -> (millisecond timer value=w5107:u32)
          }
        }
        n3900 = case shown="No Error" w5104 {
          selector: w5104 -> [w5137 w5256]
          tunnel: [w5120 w5258] -> w5105
          tunnel: [w5119 w5257] -> w5103
          tunnel: w5106 -> [w5138 w5250]
          tunnel: w5102 -> [w5118 w5249]
          tunnel: [w5117 w5249] -> w5101
          tunnel: w5100 -> [_ _]
          frame No Error {
            n3901 = Concatenate Strings("\r", "\n") -> (w5129:string)  [unwired: 1 in]
            n3902 = case shown="True" w5130 {
              tunnel: w5138 -> [w5162 w5169]
              tunnel: w5137 -> [w5161 w5168]
              tunnel: [w5162 w5167] -> w5136
              tunnel: [w5161 w5166] -> w5116
              tunnel: w5129 -> [_ w5165]
              frame False {
              }
              frame True {
                n3903 = VISA Write(VISA resource name=w5169, write buffer=w5165, error in (no error)=w5168) -> (VISA resource name out=w5167:refnum<visa-resource-name>, error out=w5166:errorcluster)  [unwired: 1 out]
                n3904 = local write "Read String"("") -> ()
                n3905 = local write item#-1(FALSE) -> ()
              }
            }
            n3906 = property class="Instr"(reference=w5136, error in=w5116) -> (reference out=w5135:refnum<visa-resource-name>, error out=w5134:errorcluster, "Serial Settings:Number of Bytes at Serial Port"=w5133:u32)
            n3907 = Greater?(x=w5133, y=u32 100) -> (0:w5131:bool)
            n3908 = case shown="True" w5131 {
              tunnel: w5135 -> [w5172 w5196]
              tunnel: w5134 -> [w5171 w5195]
              tunnel: w5133 -> [_ w5194]
              tunnel: [w5172 w5193] -> w5122
              tunnel: [w5171 w5192] -> w5121
              tunnel: w5118 -> [w5170 w5191]
              tunnel: [w5170 ""] -> w5117
              frame False {
              }
              frame True {
                w5181 = u32 6 ("y")
                # "Page 84 of \nmanual"
                n3909 = VISA Read(VISA resource name=w5196, byte count=w5194, error in (no error)=w5195) -> (VISA resource name out=w5193:refnum<visa-resource-name>, read buffer=w5189:string, error out=w5192:errorcluster)  [unwired: 1 out]
                n3910 = while {
                  tunnel: w5189 -> [w5245]
                  tunnel: [w5241] -> w5183 mode=indexing
                  tunnel: [w5235] -> w5187 mode=indexing
                  tunnel: [w5233] -> _
                  i -> [w5233]
                  stop <- w5238 stop-if-true
                  n3911 = String Subset(string=w5245, offset (0)=w5233) -> (substring=w5240:string)  [unwired: 1 in]
                  n3912 = String To Byte Array(string=w5240) -> (unsigned byte array=w5244:u8[])
                  n3913 = String Length(string=w5240) -> (length=w5239:i32)
                  n3914 = Index Array(array=w5244) -> (element=w5243:u8)  [unwired: 1 in]
                  n3915 = Equal To 0?(x=w5239) -> (x = 0?=w5238:bool)
                  n3916 = Number To Boolean Array(number=w5243) -> (Boolean array=w5237:bool[])
                  n3917 = Reverse 1D Array(array=w5237) -> (reversed array=w5236:bool[])
                  n3918 = And(x=w5237, y=bool[] [FALSE, FALSE, FALSE, FALSE, FALSE, FALSE, TRUE, TRUE] ("Boolean array")) -> (x .and. y?=w5241:bool[])
                  n3919 = And(x=w5236, y=bool[] [FALSE, FALSE, TRUE, TRUE, TRUE, TRUE, TRUE, TRUE] ("Boolean array")) -> (x .and. y?=w5235:bool[])
                }
                n3920 = Concatenate Strings(w5191, w5189) -> (→"Read String":string)
                n3921 = while {
                  tunnel: w5183 -> [w5232] mode=indexing
                  tunnel: [w5228] -> w5186
                  i -> [w5228]
                  stop <- w5229 stop-if-true
                  n3922 = Search 1D Array(1D array=w5232, element=TRUE) -> (index of element=w5230:i32)  [unwired: 1 in]
                  n3923 = Less Than 0?(x=w5230) -> (x < 0?=w5229:bool)
                }
                n3924 = Delete From Array(array=w5187, length=w5186, index (row)=0) -> (array with subset deleted=w5182:bool[][])  [unwired: 1 in, 1 out]
                n3925 = Array Size(array=w5182) -> (size(s)=w5184:i32[])
                n3926 = Index Array(array=w5184) -> (element=w5176:i32)  [unwired: 1 in]
                n3927 = Greater?(x=w5176, y=w5181) -> (0:w5179:bool)
                n3928 = Subtract(x=w5176, y=w5181) -> (x-y=w5180:u32)
                n3929 = Select(t=w5180, s=w5179, f=u32 0) -> (s? t:f=w5177:u32)
                n3930 = while {
                  tunnel: w5182 -> [w5215]
                  tunnel: [w5217] -> w5175 mode=indexing
                  tunnel: w5177 -> [w5199]
                  i -> [w5216]
                  stop <- w5214 stop-if-true
                  w5206 = 6 ("index")
                  w5205 = 2 ("length")
                  # "Page 65 of \nmanual"
                  n3931 = Multiply(x=u32 3 ("y"), y=w5216) -> (x*y=w5213:u32)
                  n3932 = Divide(x=u32 102 ("y"), y=u32 65520) -> (x/y=w5223:dbl)
                  n3933 = Greater Or Equal?(x=w5213, y=w5199) -> (x >= y?=w5214:bool)
                  n3934 = Index Array(array=w5215, index (row) #1=w5213) -> (element #1=w5211:bool[], element #2=w5210:bool[], element #3=w5209:bool[])  [unwired: 5 in]
                  n3935 = Reverse 1D Array(array=w5211) -> (reversed array=w5204:bool[])
                  n3936 = Reverse 1D Array(array=w5210) -> (reversed array=w5208:bool[])
                  n3937 = Reverse 1D Array(array=w5209) -> (reversed array=w5207:bool[])
                  n3938 = Delete From Array(array=w5204, length=w5205, index=w5206) -> (array with subset deleted=w5200:bool[])  [unwired: 1 out]
                  n3939 = Delete From Array(array=w5208, length=w5205, index=w5206) -> (array with subset deleted=w5201:bool[])  [unwired: 1 out]
                  n3940 = Delete From Array(array=w5207, length=w5205, index=w5206) -> (array with subset deleted=w5202:bool[])  [unwired: 1 out]
                  n3941 = Insert Into Array(array=bool[] [] ("Boolean array"), new element #1=w5200, new element #2=w5201, new element #3=w5202) -> (w5203:bool[])  [unwired: 1 in]
                  n3942 = Boolean Array To Number(Boolean array=w5203) -> (number=w5212:u32)
                  n3943 = Multiply(x=w5223, y=w5212) -> (x*y=w5222:dbl)
                  n3944 = Decrement(x=w5222) -> (x-1=w5221:dbl)
                  n3945 = Divide(x=w5221, y=u32 100) -> (x/y=w5219:dbl)
                  n3946 = Multiply(x=w5219, y=u32 10) -> (x*y=w5217:dbl)
                }
                n3947 = Delete From Array(array=w5175) -> (array with subset deleted=w5174:dbl[])  [unwired: 2 in, 1 out]
                "Waveform Graph 5" <- w5174
                "Waveform Chart 3" <- w5174
                n3948 = call-poly <vilib>:"Mean.vi"("X"=w5174) -> ("mean"=w5173:dbl)  [unwired: 1 out]
                n3949 = case shown="True" {
                  selector: _ -> [_ _]
                  tunnel: w5173 -> [_ w5198]
                  frame False {
                  }
                  frame True {
                    n3950 = local write item#-1(FALSE ("Zero 4")) -> ()
                    "z_measure" <- w5198
                  }
                }
              }
            }
            n3951 = local read item#-1() -> (w5113)
            n3952 = local read item#-1() -> (w5112)
            n3953 = local read item#-1() -> (w5114)
            n3954 = local read item#-1() -> (w5111)
            n3955 = case shown="True" w5109 {
              tunnel: w5113 -> [_ w5141]
              tunnel: w5114 -> [_ w5140]
              frame False {
              }
              frame True {
                n3956 = Build Array(w5141, w5140) -> (w5139:void[])
                n3957 = local read item#-1() -> (w5144)
                n3958 = Build Array (concatenate)(w5144, w5139) -> (w5142:void[])
                n3959 = local write item#-1(w5142) -> ()
                n3960 = local write item#-1(FALSE ("Boolean 8")) -> ()
              }
            }
            n3961 = call "Build XY Graph"("Enable"=w5111, "Reset"=w5112, "Y Input"=w5114, "X Input"=w5113) -> ("XY Graph"=w5110:cluster{"Y":dbl[], "Y":dbl[]}[])  [unwired: 6 in, 1 out]
            n3962 = case shown="True" {
              selector: _ -> [_ _]
              frame False {
              }
              frame True {
                n3963 = local read item#-1() -> (w5145)
                n3964 = Index Array(array=w5145, index (col) #1=0 ("disabled index (col)"), index (col) #2=1 ("index (col)")) -> (element #1=w5147, element #2=w5146)  [unwired: 2 in]
                n3965 = call <vilib>:"Linear Fit.vi"("Y"=w5147, "X"=w5146) -> ()  [unwired: 9 in, 5 out]
                n3966 = local write item#-1(FALSE ("Boolean 9")) -> ()
              }
            }
            n3967 = case shown="True" {
              selector: _ -> [_ _]
              frame False {
              }
              frame True {
                n3968 = local write item#-1(dbl[][] [] ("Captured Values")) -> ()
                n3969 = local write item#-1(FALSE ("Boolean 7")) -> ()
              }
            }
            n3970 = Concatenate Strings("\r", "\n") -> (w5124:string, w5123:string)
            n3971 = case shown="True" w5115 {
              tunnel: w5122 -> [w5154 w5160]
              tunnel: w5121 -> [w5153 w5159]
              tunnel: [w5154 w5158] -> w5120
              tunnel: [w5153 w5157] -> w5119
              tunnel: w5124 -> [_ w5156]
              frame False {
              }
              frame True {
                n3972 = VISA Write(VISA resource name=w5160, write buffer=w5156, error in (no error)=w5159) -> (VISA resource name out=w5158:refnum<visa-resource-name>, error out=w5157:errorcluster)  [unwired: 1 out]
                n3973 = local write item#-1(FALSE ("WRITE")) -> ()
              }
            }
          }
          frame Error {
            w5248 = u16 10 items=["1.0"=10, "1.5"=15, "2.0"=20] ("stop bits (10: 1 bit)")
            n3974 = Wait (ms)(milliseconds to wait=u32 20) -> ()  [unwired: 1 out]
            n3975 = VISA Close(VISA resource name=w5250, error in (no error)=w5256) -> (error out=w5255:errorcluster)
            n3976 = call <vilib>:"Clear Errors.vi"("error in (no error)"=w5255) -> ("error out"=w5254:errorcluster)  [unwired: 5 in, 1 out]
            n3977 = call-poly "VISA Configure Serial Port"("timeout (10sec)"=u32 200, "Enable Termination\nChar (T)"=TRUE ("Enable Termination\nChar (T)"), "baud rate (9600)"=u32 921600, "error in (no error)"=w5254, "stop bits (10: 1 bit)"=w5248) -> ("VISA resource name"=w5246:refnum<visa-resource-name>, "VISA resource name out"=w5258:refnum<visa-resource-name>, "error out"=w5257:errorcluster)  [unwired: 8 in]
          }
        }
        n3978 = local read "Quit"() -> (w5098:bool)
      }
      n3979 = VISA Close(VISA resource name=w5093, error in (no error)=w5094) -> (error out=w5092:errorcluster)
      n3980 = call <vilib>:"Clear Errors.vi"("error in (no error)"=w5092) -> ()  [unwired: 5 in, 2 out]
    }
    frame Enabled {
    }
  }
  n3981 = disable-structure shown="Disabled" {
    disable-tunnel: _ -> [w5263 _]
    frame Disabled {
      n3982 = while {
        tunnel: [w5270] -> _
        shift-right: [w5267] -> w5260
        shift-left: _ -> [w5269]
        shift-right: [w5268] -> w5261
        shift-left: errorcluster {"status"=TRUE, "code"=0, "source"="Init"} ("error out") -> [w5266]
        tunnel: w5263 -> [_]
        i -> [w5270]
        stop <- w5264 stop-if-true
        n3983 = flat-sequence {
          tunnel: w5266 -> [w5361]
          tunnel: [w5361] -> w5265
          frame #0 {
            n3984 = Wait (ms)(milliseconds to wait=u32 50) -> ()  [unwired: 1 out]
          }
        }
        n3985 = case shown="No Error" w5265 {
          selector: w5265 -> [w5311 w5354]
          tunnel: w5269 -> [w5310 w5353]
          tunnel: [w5277 w5344] -> w5268
          tunnel: [w5278 w5352] -> w5267
          frame No Error {
            w5304 = T32 {"Mode"=enum."RTU", "Slave Address"=1} ("Serial Parameters")
            n3986 = call-poly <vilib>:"MB Serial Master Query (poly).vi"("VISA resource name"=w5310, "Starting Address"=i16 1000, "Quantity"=u16 1, "Timeout"=u32 1000, "error in"=w5311, "Serial Parameters"=w5304) -> ("VISA resource name out"=w5305:refnum<visa-resource-name>, "Input Registers"=w5307:u16[], "error out"=w5303:errorcluster)  [unwired: 10 in, 1 out]
            n3987 = Random Number (0-1)() -> (number: 0 to 1=w5292:dbl)
            n3988 = Index Array(array=w5307, index=0) -> (element=w5302:u16)
            n3989 = Subtract(x=w5292, y=0.5) -> (x-y=w5291:dbl)
            n3990 = Divide(x=w5302, y=10 ("index")) -> (x/y=w5296:dbl)
            n3991 = Multiply(x=w5291, y=0.5) -> (x*y=w5290:dbl)
            n3992 = Add(x=w5296, y=w5290) -> (x+y=w5295:dbl)
            n3993 = local read "Amb temp"() -> (w5279:dbl)
            n3994 = Multiply(x=w5295, y=0.2) -> (x*y=w5299:dbl)
            n3995 = Multiply(x=w5279, y=0.8) -> (x*y=w5297:dbl)
            n3996 = Add(x=w5299, y=w5297) -> (x+y=w5280:dbl)
            n3997 = local read "set temp old"() -> (w5274:dbl)
            n3998 = local write "Amb temp"(w5280) -> ()
            n3999 = Select(t="SetTemp 2", s="Heater", f=100.0) -> (s? t:f=w5275:dbl)
            n4000 = Not Equal?(x=w5275, y=w5274) -> (x != y?=w5273:bool)
            n4001 = case shown="True" w5273 {
              tunnel: w5305 -> [w5339 w5341]
              tunnel: [w5338 w5341] -> w5285
              tunnel: w5303 -> [w5337 w5340]
              tunnel: [w5336 w5340] -> w5283
              tunnel: w5275 -> [w5331 _]
              tunnel: w5304 -> [w5333 w5342]
              tunnel: [w5333 w5342] -> w5286
              frame True {
                n4002 = Multiply(x=w5331, y=10 ("index")) -> (x*y=w5330:dbl)
                n4003 = call-poly <vilib>:"MB Serial Master Query (poly).vi"("VISA resource name"=w5339, "Address"=u16 0, "Holding Register"=w5330, "Timeout"=u32 1000, "error in"=w5337, "Serial Parameters"=w5333) -> ("VISA resource name out"=w5338:refnum<visa-resource-name>, "error out"=w5336:errorcluster)  [unwired: 11 in, 1 out]
                "set temp old" <- w5331
              }
              frame False {
              }
            }
            n4004 = flat-sequence {
              tunnel: [w5312] -> _
              tunnel: [w5312] -> w5282
              tunnel: w5283 -> [w5312]
              frame #0 {
                n4005 = Wait (ms)(milliseconds to wait=u32 100) -> ()  [unwired: 1 out]
              }
            }
            n4006 = call "Elapsed Time12"("Time Target (s)"=2.0, "Auto Reset"=TRUE) -> ("Time has Elapsed"=w5287:bool)  [unwired: 10 in, 7 out]
            n4007 = case shown="True" w5287 {
              tunnel: w5286 -> [w5316 w5329]
              tunnel: [w5316 w5329] -> _
              tunnel: [w5315 w5327] -> w5278
              tunnel: w5285 -> [w5315 w5328]
              tunnel: [w5314 w5325] -> w5277
              tunnel: w5282 -> [w5314 w5326]
              frame False {
              }
              frame True {
                n4008 = call-poly <vilib>:"MB Serial Master Query (poly).vi"("VISA resource name"=w5328, "Starting Address"=i16 1003 ("Addr"), "Quantity"=u16 1, "Timeout"=u32 1000, "error in"=w5326, "Serial Parameters"=w5329) -> ("VISA resource name out"=w5327:refnum<visa-resource-name>, "Input Registers"=w5322:u16[], "error out"=w5325:errorcluster)  [unwired: 10 in, 1 out]
                n4009 = Index Array(array=w5322, index=0) -> (element=w5321:u16)
                n4010 = Divide(x=w5321, y=u16 10) -> (x/y=w5317:dbl)
                n4011 = local write "set temp old"(w5317) -> ()
                n4012 = local write "SetTemp"(w5317) -> ()
              }
            }
            "Error Code" <- w5277
            n4013 = Unbundle(w5277) -> ("status"=→"TK4 status":bool)  [unwired: 2 out]
            "SetTemp" <- "SetTemp 2"
          }
          frame Error {
            w5356 = u16 0 items=["None", "Odd", "Even", "Mark", "Space"] ("Parity")
            w5357 = u16 0 items=["None", "XON/XOFF", "RTS/CTS", "XON/XOFF & RTS/CTS", "DTR/DSR", "XON/XOFF & DTR/DSR"] ("Flow Control")
            n4014 = VISA Clear(VISA resource name=w5353, error in (no error)=w5354) -> (VISA resource name out=w5347:refnum<visa-resource-name>, error out=w5345:errorcluster)
            n4015 = VISA Close(VISA resource name=w5347, error in (no error)=w5345) -> (error out=w5346:errorcluster)
            n4016 = call <vilib>:"Clear Errors.vi"("error in (no error)"=w5346) -> ("error out"=w5355:errorcluster)  [unwired: 5 in, 1 out]
            n4017 = Unbundle By Name(T32 {"Mode"=enum."RTU", "Slave Address"=1} ("input cluster")) -> ("Mode"=w5358:enum16{"RTU", "ASCII"})
            n4018 = call <vilib>:"MB Serial Init.vi"("Timeout"=u32 100, "Flow Control"=w5357, "Mode"=w5358, "error in (no error)"=w5355, "Parity"=w5356, "Baud Rate"=u32 9600, "VISA resource name"="Lubrication System COM Port :") -> ("error out"=w5344:errorcluster, "VISA resource name out"=w5352:refnum<visa-resource-name>)  [unwired: 3 in]
            n4019 = local write "set temp old"(0.0 ("set temp old")) -> ()
